vi "Assert Map to Array Round Trip.vi"(7 "Label":string="Map to Array (Round Trip)", 8 "error in (no error)":errorcluster, 11 "Variant":variant) -> (0 "error out":errorcluster, 2 "Passed":bool)   [LabVIEW 2020]
uses:
  source/library/Get Collection Subtype.vi
  <vilib>/addons/_JKI Toolkits/Caraya/classes/Assert/Assert.lvclass
  source/library/openg_variant.lvlib
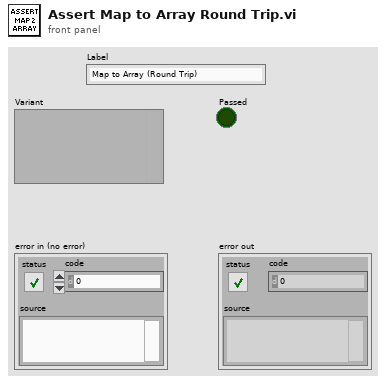
[diagram p1: front panel]
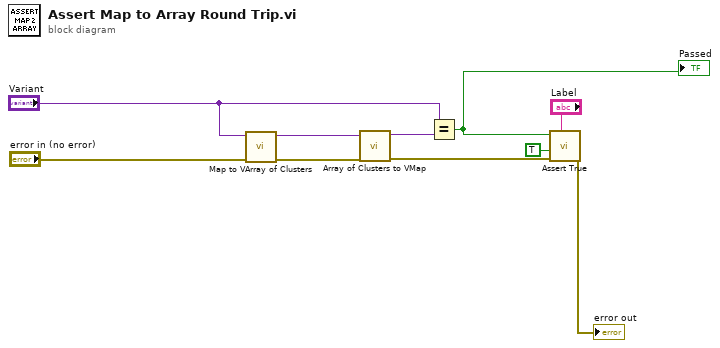
[diagram p0: block diagram]
diagram:
  n1 = call "Map to VArray of Clusters.vi"("error in"="error in (no error)", "Map"="Variant") -> ("error out"=w7:errorcluster, "Array of Clusters (key-value)"=w4:variant)  [unwired: 8 in]
  n2 = call "Array of Clusters to VMap.vi"("error in"=w7, "Array of Clusters (key-value)"=w4) -> ("error out"=w8:errorcluster, "Map"=w5:variant)  [unwired: 8 in]
  n3 = Equal?(x="Variant", y=w5) -> (x = y?=w6:bool)
  "Passed" <- w6
  n4 = call <vilib>:"Assert True.vi"("Label"="Label", "error in (no error)"=w8, "Register with caller test (F)"=TRUE, "True?"=w6) -> ("error out"=→"error out":errorcluster)  [unwired: 7 in]
